vi "Set Distance Type.vi"(8 "error in (no error)":errorcluster, 9 "Minkowsky Order":i32=1, 10 "distance type":T1=1 items=["EUCLIDEAN"=1, "MANHATTAN"=2, "MINKOWSKY"=3, "HIST INTERSECT"=5, "HELLINGER"=6, "CHI SQUARE"=7, "KULLBACK LEIBLER"=8], 11 "KD Tree in":refnum<class "KD Tree.lvclass">) -> (0 "error out":errorcluster, 3 "KD Tree out":refnum<class "KD Tree.lvclass">)   [LabVIEW 2020, in "KD Tree.lvlib" / "KD Tree.lvclass"]
uses:
  KD Tree.lvclass
  KD Tree.lvlib
  Wrapper/Distance Type.ctl
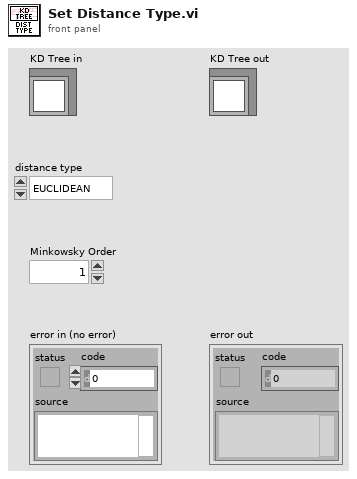
[diagram p1: front panel]
types:
  T1 = typedef "KD Tree.lvlib/Distance Type.ctl" = u32
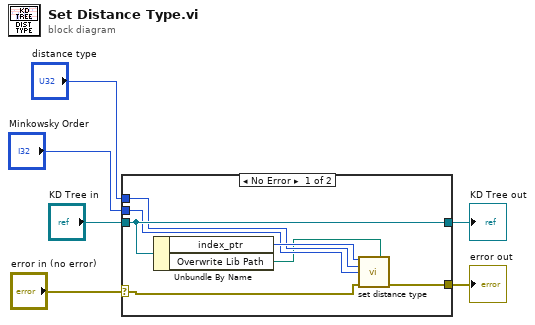
[diagram p0: block diagram]
diagram:
  n1 = case shown="No Error" "error in (no error)" {
    selector: "error in (no error)" -> [w11 w15]
    tunnel: [w7 w15] -> w5
    tunnel: [w13 w14] -> w3
    tunnel: "KD Tree in" -> [w13 w14]
    tunnel: "distance type" -> [w10 _]
    tunnel: "Minkowsky Order" -> [w9 _]
    frame No Error {
      n2 = Unbundle By Name(w13) -> ("index_ptr"=w12:u64, "Overwrite Lib Path"=w8:path)
      n3 = call "set distance type.vi"("index_id"=w12, "Overwrite Lib Path"=w8, "distance type"=w10, "Minkowsky Order"=w9, "error in (no error)"=w11) -> ("error out"=w7:errorcluster)  [unwired: 9 in, 1 out]
    }
    frame Error {
    }
  }
  "error out" <- w5
  "KD Tree out" <- w3
